vi "Search Key Name Array.vi"(10 "Key Name":string, 11 "Keys":refnum<class "Key Name.lvclass">[](array[class])) -> (1 "Found?":bool, 2 "Index":i32, 3 "Keys dup":refnum<class "Key Name.lvclass">[](array[class]))   [LabVIEW 2019, in "Electronic Datasheet.lvlib" / "Key Name.lvclass"]
uses:
  Key Name.lvclass
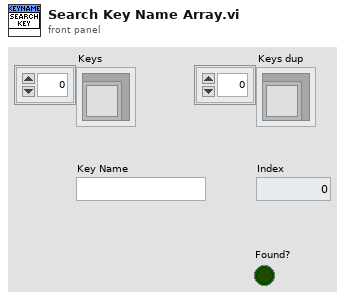
[diagram p1: front panel]
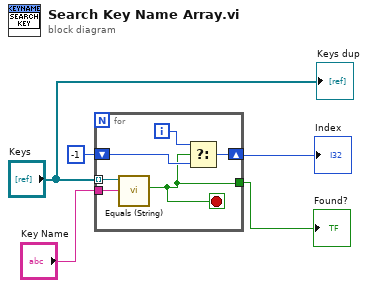
[diagram p0: block diagram]
diagram:
  n1 = for {
    tunnel: "Keys" -> [w8] mode=indexing
    tunnel: "Key Name" -> [w7]
    shift-right: [w11] -> w3
    shift-left: -1 -> [w9]
    tunnel: [w6] -> w1
    i -> [w10]
    stop <- w6 stop-if-true
    n2 = call "Equals (String).vi"("Keyname"=w7, "Keyname in"=w8) -> ("Equal?"=w6:bool)  [unwired: 8 in, 1 out]
    n3 = Select(t=w10, s=w6, f=w9) -> (s? t:f=w11:i32)
  }
  "Index" <- w3
  "Found?" <- w1
  "Keys dup" <- "Keys"
